vi "Update Animation.vi"(11 "Asteroid in":refnum<class "Asteroid.lvclass">) -> (3 "Asteroid out":refnum<class "Asteroid.lvclass">)   [LabVIEW 2021, in "Asteroid.lvclass"]
uses:
  Asteroid.lvclass
  Asteroid.lvclass/Asteroid.ctl
  <userlib>/_OpenG.lib/boolean/boolean.llb/openg_boolean__ogtk.lvlib
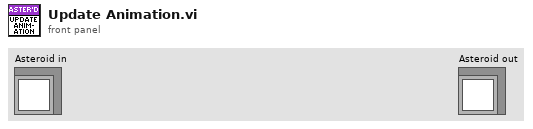
[diagram p1: front panel]
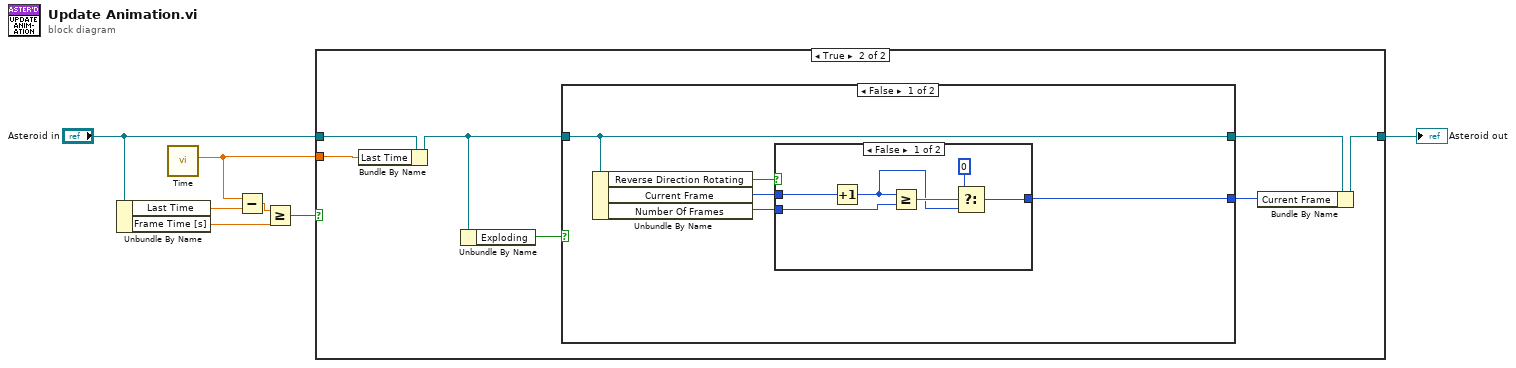
[diagram p0: block diagram]
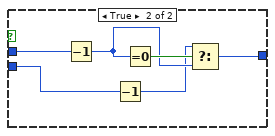
[diagram p3: hidden frame]
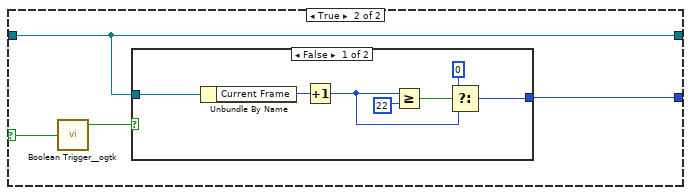
[diagram p4: hidden frame]
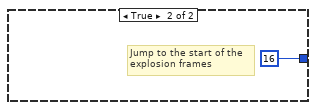
[diagram p5: hidden frame]
diagram:
  n1 = Unbundle By Name("Asteroid in") -> ("Last Time"=w5:sgl, "Frame Time [s]"=w3:sgl)
  n2 = call "Time.vi"() -> ("Time [s]"=w1:sgl)  [unwired: 10 in, 1 out]
  n3 = Subtract(x=w1, y=w5) -> (x-y=w4:sgl)
  n4 = Greater Or Equal?(x=w4, y=w3) -> (x >= y?=w7:bool)
  n5 = case shown="True" w7 {
    tunnel: [w8 w11] -> w2
    tunnel: "Asteroid in" -> [w8 w14]
    tunnel: w1 -> [_ w12]
    frame False {
    }
    frame True {
      n6 = Bundle By Name(cluster=w14, "Last Time"=w12) -> (w13:refnum<class "Asteroid.lvclass">)
      n7 = Unbundle By Name(w13) -> ("Exploding"=w15:bool)
      n8 = case shown="False" w15 {
        selector: w15 -> [_ w36]
        tunnel: [w18 w33] -> w10
        tunnel: w13 -> [w18 w33]
        tunnel: [w17 w34] -> w9
        frame False {
          n9 = Unbundle By Name(w18) -> ("Reverse Direction Rotating"=w16:bool, "Current Frame"=w20:i32, "Number Of Frames"=w19:i32)
          n10 = case shown="False" w16 {
            tunnel: w20 -> [w26 w32]
            tunnel: w19 -> [w25 w28]
            tunnel: [w21 w30] -> w17
            frame False {
              n11 = Increment(x=w26) -> (x+1=w22:i32)
              n12 = Greater Or Equal?(x=w22, y=w25) -> (x >= y?=w24:bool)
              n13 = Select(t=0, s=w24, f=w22) -> (s? t:f=w21:i32)
            }
            frame True {
              n14 = Decrement(x=w32) -> (x-1=w29:i32)
              n15 = Decrement(x=w28) -> (x-1=w27:i32)
              n16 = Equal To 0?(x=w29) -> (x = 0?=w31:bool)
              n17 = Select(t=w27, s=w31, f=w29) -> (s? t:f=w30:i32)
            }
          }
        }
        frame True {
          n18 = call <userlib>:"Boolean Trigger__ogtk.vi"("Boolean Input"=w36) -> ("Rising Edge"=w35:bool)  [unwired: 1 in, 1 out]
          n19 = case shown="False" w35 {
            tunnel: [w42 16 ("t")] -> w34
            tunnel: w33 -> [w37 _]
            frame False {
              n20 = Unbundle By Name(w37) -> ("Current Frame"=w43:i32)
              n21 = Increment(x=w43) -> (x+1=w39:i32)
              n22 = Greater Or Equal?(x=w39, y=22) -> (x >= y?=w41:bool)
              n23 = Select(t=0, s=w41, f=w39) -> (s? t:f=w42:i32)
            }
            frame True {
              # "Jump to the start of the explosion frames"
            }
          }
        }
      }
      n24 = Bundle By Name(cluster=w10, "Current Frame"=w9) -> (w11:refnum<class "Asteroid.lvclass">)
    }
  }
  "Asteroid out" <- w2
